vi "startwlm.vi"   [LabVIEW 2014]
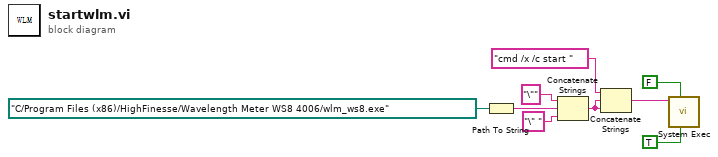
[diagram p0: block diagram]
diagram:
  n1 = Path To String(path=path "C:/Program Files (x86)/HighFinesse/Wavelength Meter WS8 4006/wlm_ws8.exe" ("file path (use dialog)")) -> (string=w7:string)
  n2 = Concatenate Strings("\"", w7, "\" ") -> (w2:string)
  n3 = Concatenate Strings("cmd /x /c start " ("string"), w2, w2) -> (w5:string)
  n4 = call <vilib>:"System Exec.vi"("run minimized? (F)"=TRUE, "wait until completion? (T)"=FALSE, "command line"=w5) -> ()  [unwired: 5 in, 4 out]
